vi "Get Range.vi"(0 "object in":refnum<class "HPS-17000-PowerModule.lvclass">, 11 "Error In":errorcluster) -> (4 "object out":refnum<class "HPS-17000-PowerModule.lvclass">, 6 "Range":T1, 15 "Error Out":errorcluster)   [LabVIEW 2023, in "HPS-17000-PowerModule.lvlib" / "HPS-17000-PowerModule.lvclass"]
uses:
  HPS-17000-PowerModule.lvclass
  builds/PowerModuleInterface/PowerModuleInterface.lvlibp/Classes/PowerModule_interface/Range.ctl
  <instrlib>/HPS-17000/Client Facing Datatypes/Range.ctl
  <instrlib>/HPS-17000/Internal/Get Mode Multi.vi
  <instrlib>/HPS-17000/HPS-17000.lvclass
  builds/PowerModuleInterface/PowerModuleInterface.lvlibp/Classes/PowerModule_interface/PowerModuleInterface.lvclass
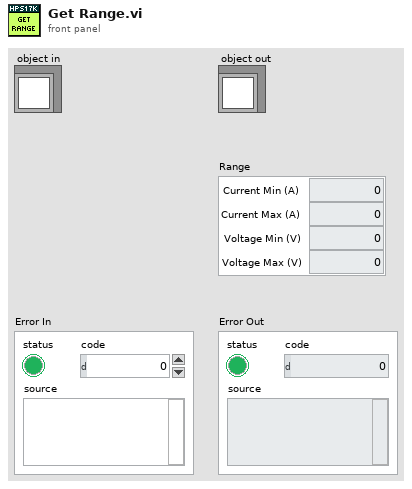
[diagram p1: front panel]
types:
  T1 = typedef "PowerModuleInterface.lvlibp/PowerModuleInterface.lvclass/Range.ctl" = cluster{"Current Max (A)":dbl, "Current Min (A)":dbl, "Voltage Max (V)":dbl, "Voltage Min (V)":dbl}
  T2 = typedef "HPS-17000-PowerModule.lvlib/HPS-17000-PowerModule.lvclass/ObjectAttributes.ctl" = cluster{"JSON Config Path":path, "Configuration":T3, "GM ID":string, "HPS17000 Refs":refnum<class "HPS-17000.lvclass">[], "connected":bool, "reserved":bool, "events":T5, "nibatterycycler_grpc_Setpoint":T6, "last timestamp":i64, "mode":T7, "range":T1, "measurement array":T8[]}
  T3 = typedef "HPS-17000-PowerModule.lvlib/HPS-17000-PowerModule.lvclass/Configuration.ctl" = cluster{"TSN NIC IP Address":string, "HPS17000 IP Addresses":string[], "HPS Topology":enum16{"SINGLE", "MULTI"}, "Setpoint Stream Config":T4, "Measurement Array Size":i32}
  T4 = typedef "Cycler.lvclass/Setpoint Stream Basic Config.ctl" = cluster{"local address":string, "receiver port":u16}
  T5 = typedef "HPS-17000.lvclass/Multi-Cycler Events.ctl" = cluster{"heartbeats events":refnum<user-event>[], "faults events":refnum<user-event>[], "network sync event":refnum<user-event>[], "setpoint status event":refnum<user-event>[]}
  T6 = typedef "NI_BC_client.lvlib/nibatterycycler_grpc_Setpoint.ctl" = cluster{"voltage":sgl, "current":sgl, "min_power":sgl, "max_power":sgl, "resistance":sgl}
  T7 = typedef "HPS-17000-PowerModule.lvlib/HPS-17000-PowerModule.lvclass/Mode.ctl" = u16
  T8 = typedef "PowerModuleInterface.lvlibp/PowerModuleInterface.lvclass/Measurements.ctl" = cluster{"measured voltage (V)":dbl, "measured current (A)":dbl, "setpoint voltage (V)":dbl, "setpoint current (A)":dbl, "timestamp":dbl}
  T9 = typedef "HPS-17000.lvclass/Range.ctl" = u8
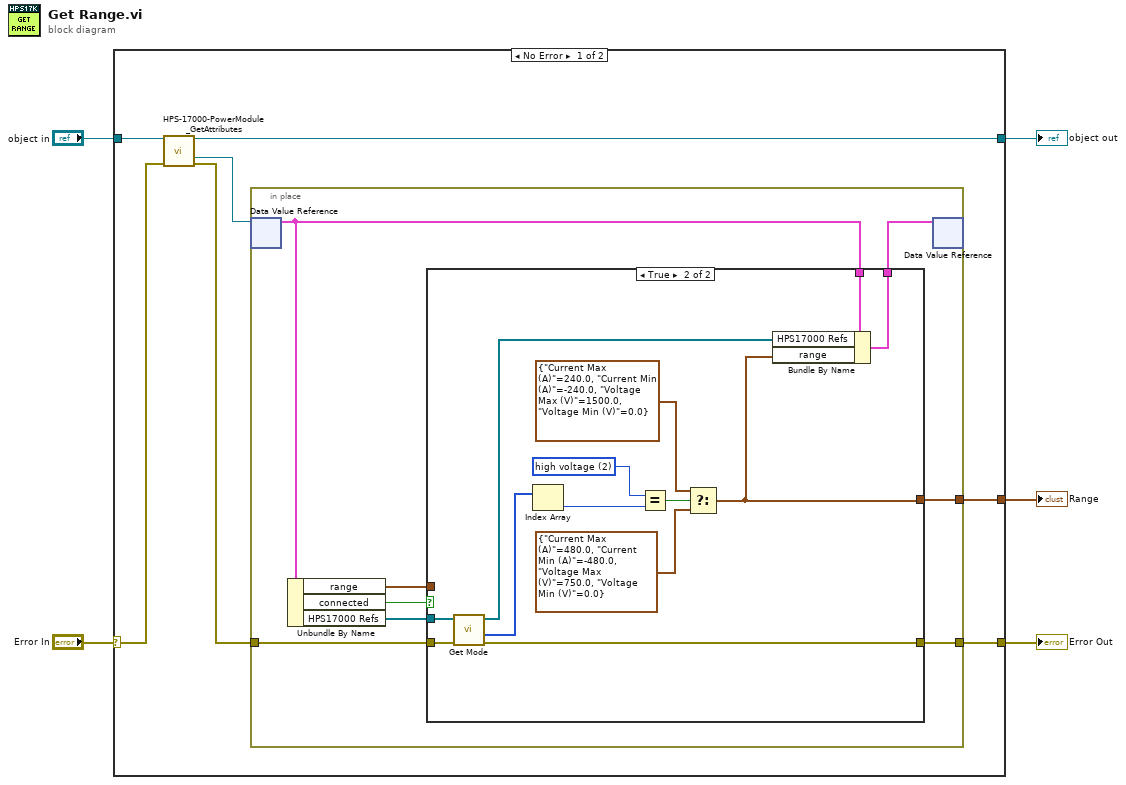
[diagram p0: block diagram]
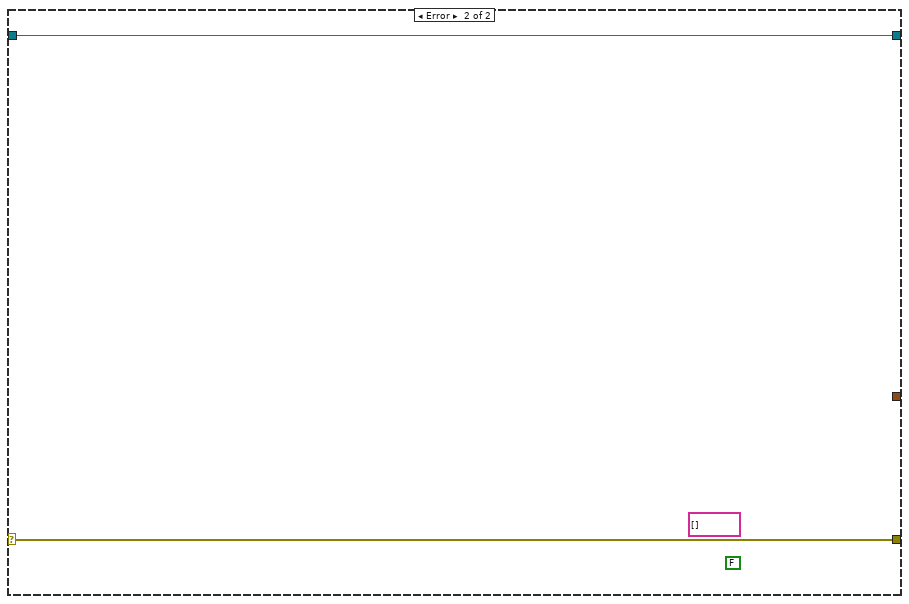
[diagram p3: hidden frame]
diagram:
  n1 = case shown="No Error" "Error In" {
    selector: "Error In" -> [w11 w37]
    tunnel: "object in" -> [w12 w38]
    tunnel: [w7 w38] -> w3
    tunnel: [w8 w37] -> w2
    tunnel: [w6 _] -> w1
    frame No Error {
      n2 = call "HPS-17000-PowerModule_GetAttributes.vi"("reference in"=w12, "Error In"=w11) -> ("reference out"=w7:refnum<class "HPS-17000-PowerModule.lvclass">, "DataRef"=w10:refnum<data-value>, "Error Out"=w9:errorcluster)  [unwired: 10 in, 1 out]
      n3 = in-place {
        in-place-border: w9 -> [w18]
        in-place-border: [w17] -> w8
        in-place-border: [w14] -> w6
        n4 = in-place-dvr #1(w10) -> (w19:T2)  [unwired: 1 out]
        n5 = Unbundle By Name(w19) -> ("range"=w13:T1, "connected"=w15:bool, "HPS17000 Refs"=w16:refnum<class "HPS-17000.lvclass">[])
        n6 = case shown="True" w15 {
          tunnel: [w23 w36] -> w20
          tunnel: w19 -> [w23 w35]
          tunnel: w18 -> [w22 w34]
          tunnel: [w22 w30] -> w17
          tunnel: w16 -> [_ w33]
          tunnel: [w21 w24] -> w14
          tunnel: w13 -> [w21 _]
          frame False {
          }
          frame True {
            w28 = T9 2 items=["low voltage"=1, "high voltage"=2] ("element")
            n7 = call-poly <instrlib>:"Get Mode.vi"("error in"=w34, "cycler refs in"=w33) -> ("error out"=w30:errorcluster, "range"=w31:T9[], "cycler refs out"=w32:refnum<class "HPS-17000.lvclass">[])  [unwired: 6 in, 1 out]
            n8 = Index Array(array=w31) -> (element=w29:T9)  [unwired: 1 in]
            n9 = Equal?(x=w28, y=w29) -> (x = y?=w27:bool)
            n10 = Select(t=T1 {"Current Max (A)"=240.0, "Current Min (A)"=-240.0, "Voltage Max (V)"=1500.0, "Voltage Min (V)"=0.0} ("range"), s=w27, f=T1 {"Current Max (A)"=480.0, "Current Min (A)"=-480.0, "Voltage Max (V)"=750.0, "Voltage Min (V)"=0.0} ("range")) -> (s? t:f=w24:T1)
            n11 = Bundle By Name(cluster=w35, "HPS17000 Refs"=w32, "range"=w24) -> (w36:T2)
          }
        }
        n12 = in-place-dvr #1(w20) -> ()  [unwired: 2 out]
      }
    }
    frame Error {
      (unwired) string[] []
      (unwired) FALSE
    }
  }
  "Error Out" <- w2
  "object out" <- w3
  "Range" <- w1
